vi "Toggle Debugging_Item_OnCommand.vi"(10 "Command ID":string, 11 "Object":T1) -> ()   [LabVIEW 2019]
uses:
  <resource>/Framework/Providers/API/ItemRef.ctl
panel:
  out "error out":errorcluster
  in  "error in":errorcluster
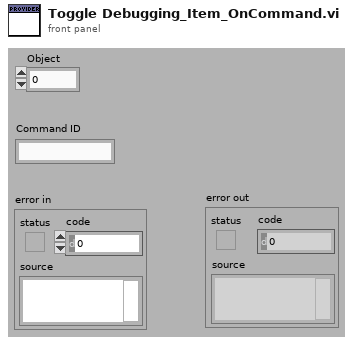
[diagram p1: front panel]
types:
  T1 = typedef "ItemRef.ctl" = u64
  T2 = enum32{"Invalid", "Standard", "Closed", "Hidden", "Minimized", "Maximized"}
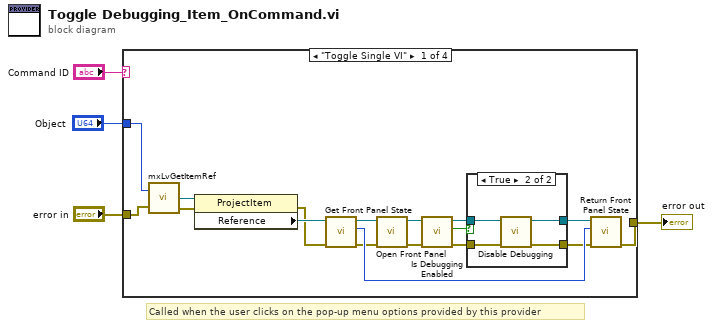
[diagram p0: block diagram]
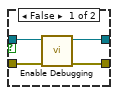
[diagram p2: hidden frame]
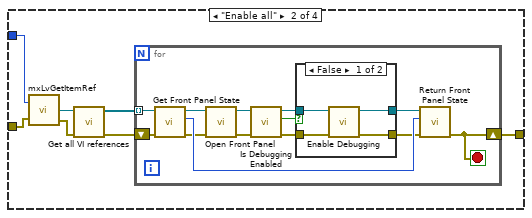
[diagram p3: hidden frame]
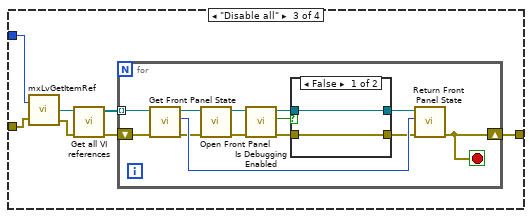
[diagram p5: hidden frame]
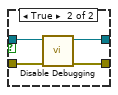
[diagram p6: hidden frame]
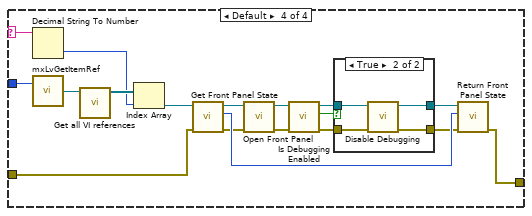
[diagram p7: hidden frame]
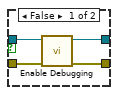
[diagram p8: hidden frame]
diagram:
  # "Called when the user clicks on the pop-up menu options provided by this provider"
  n1 = case shown="\"Toggle Single VI\"" "Command ID" {
    selector: "Command ID" -> [_ _ _ w99]
    tunnel: "error in" -> [w17 w32 w58 w83]
    tunnel: [w5 w30 w56 w82] -> w3
    tunnel: "Object" -> [w21 w35 w61 w98]
    frame "Toggle Single VI" {
      n2 = call <resource>:"mxLvGetItemRef.vi"("Item"=w21, "error in"=w17) -> ("Item Refnum"=w20:refnum<vi>, "error out"=w16:errorcluster)  [unwired: 1 out]
      n3 = property class="ProjectItem"(reference=w20, error in=w16) -> (error out=w8:errorcluster, "Reference"=w13:refnum<vi>)  [unwired: 1 out]
      n4 = call "Get Front Panel State.vi"("error in (no error)"=w8, "reference"=w13) -> ("error out"=w7:errorcluster, "Front Panel Window State"=w10:T2, "reference out"=w12:refnum<vi>)  [unwired: 7 in]
      n5 = call "Open Front Panel.vi"("error in (no error)"=w7, "reference"=w12) -> ("error out"=w6:errorcluster, "reference out"=w14:refnum<vi>)  [unwired: 8 in]
      n6 = call "Is Debugging Enabled.vi"("error in (no error)"=w6, "VI Reference In"=w14) -> ("error out"=w15:errorcluster, "Debugging Enabled?"=w19:bool, "VI Reference Out"=w18:refnum<vi>)  [unwired: 7 in]
      n7 = case shown="True" w19 {
        tunnel: w18 -> [w25 w29]
        tunnel: w15 -> [w24 w28]
        tunnel: [w23 w27] -> w9
        tunnel: [w22 w26] -> w11
        frame False {
          n8 = call "Enable Debugging.vi"("error in (no error)"=w24, "VI Reference In"=w25) -> ("error out"=w23:errorcluster, "VI Reference Out"=w22:refnum<vi>)  [unwired: 8 in]
        }
        frame True {
          n9 = call "Disable Debugging.vi"("error in (no error)"=w28, "VI Reference In"=w29) -> ("error out"=w27:errorcluster, "VI Reference Out"=w26:refnum<vi>)  [unwired: 8 in]
        }
      }
      n10 = call "Return Front Panel State.vi"("error in (no error)"=w9, "State"=w10, "reference"=w11) -> ("error out"=w5:errorcluster)  [unwired: 7 in, 1 out]
    }
    frame "Enable all" {
      n11 = call <resource>:"mxLvGetItemRef.vi"("Item"=w35, "error in"=w32) -> ("Item Refnum"=w36:refnum<vi>, "error out"=w33:errorcluster)  [unwired: 1 out]
      n12 = call "Get all VI references.vi"("error in (no error)"=w33, "Project Item"=w36) -> ("error out"=w31:errorcluster, "VI Refs"=w34:refnum<vi>[])  [unwired: 8 in]
      n13 = for {
        tunnel: w34 -> [w39] mode=indexing
        shift-right: [w37] -> w30
        shift-left: w31 -> [w38]
        stop <- w37 stop-if-true
        n14 = call "Get Front Panel State.vi"("error in (no error)"=w38, "reference"=w39) -> ("error out"=w41:errorcluster, "Front Panel Window State"=w43:T2, "reference out"=w45:refnum<vi>)  [unwired: 7 in]
        n15 = call "Open Front Panel.vi"("error in (no error)"=w41, "reference"=w45) -> ("error out"=w40:errorcluster, "reference out"=w46:refnum<vi>)  [unwired: 8 in]
        n16 = call "Is Debugging Enabled.vi"("error in (no error)"=w40, "VI Reference In"=w46) -> ("error out"=w47:errorcluster, "Debugging Enabled?"=w49:bool, "VI Reference Out"=w48:refnum<vi>)  [unwired: 7 in]
        n17 = case shown="False" w49 {
          tunnel: w48 -> [w53 w55]
          tunnel: w47 -> [w52 w54]
          tunnel: [w51 w54] -> w42
          tunnel: [w50 w55] -> w44
          frame False {
            n18 = call "Enable Debugging.vi"("error in (no error)"=w52, "VI Reference In"=w53) -> ("error out"=w51:errorcluster, "VI Reference Out"=w50:refnum<vi>)  [unwired: 8 in]
          }
          frame True {
          }
        }
        n19 = call "Return Front Panel State.vi"("error in (no error)"=w42, "State"=w43, "reference"=w44) -> ("error out"=w37:errorcluster)  [unwired: 7 in, 1 out]
      }
    }
    frame "Disable all" {
      n20 = call <resource>:"mxLvGetItemRef.vi"("Item"=w61, "error in"=w58) -> ("Item Refnum"=w62:refnum<vi>, "error out"=w59:errorcluster)  [unwired: 1 out]
      n21 = call "Get all VI references.vi"("error in (no error)"=w59, "Project Item"=w62) -> ("error out"=w57:errorcluster, "VI Refs"=w60:refnum<vi>[])  [unwired: 8 in]
      n22 = for {
        tunnel: w60 -> [w65] mode=indexing
        shift-right: [w63] -> w56
        shift-left: w57 -> [w64]
        stop <- w63 stop-if-true
        n23 = call "Get Front Panel State.vi"("error in (no error)"=w64, "reference"=w65) -> ("error out"=w67:errorcluster, "Front Panel Window State"=w69:T2, "reference out"=w71:refnum<vi>)  [unwired: 7 in]
        n24 = call "Open Front Panel.vi"("error in (no error)"=w67, "reference"=w71) -> ("error out"=w66:errorcluster, "reference out"=w72:refnum<vi>)  [unwired: 8 in]
        n25 = call "Is Debugging Enabled.vi"("error in (no error)"=w66, "VI Reference In"=w72) -> ("error out"=w73:errorcluster, "Debugging Enabled?"=w75:bool, "VI Reference Out"=w74:refnum<vi>)  [unwired: 7 in]
        n26 = case shown="False" w75 {
          tunnel: w74 -> [w77 w81]
          tunnel: w73 -> [w76 w80]
          tunnel: [w76 w79] -> w68
          tunnel: [w77 w78] -> w70
          frame False {
          }
          frame True {
            n27 = call "Disable Debugging.vi"("error in (no error)"=w80, "VI Reference In"=w81) -> ("error out"=w79:errorcluster, "VI Reference Out"=w78:refnum<vi>)  [unwired: 8 in]
          }
        }
        n28 = call "Return Front Panel State.vi"("error in (no error)"=w68, "State"=w69, "reference"=w70) -> ("error out"=w63:errorcluster)  [unwired: 7 in, 1 out]
      }
    }
    frame Default {
      n29 = Decimal String To Number(string=w99) -> (number=w95:i32)  [unwired: 2 in, 1 out]
      n30 = call <resource>:"mxLvGetItemRef.vi"("Item"=w98) -> ("Item Refnum"=w97:refnum<vi>)  [unwired: 1 in, 2 out]
      n31 = call "Get all VI references.vi"("Project Item"=w97) -> ("VI Refs"=w96:refnum<vi>[])  [unwired: 9 in, 1 out]
      n32 = Index Array(array=w96, index=w95) -> (element=w84:refnum<vi>)
      n33 = call "Get Front Panel State.vi"("error in (no error)"=w83, "reference"=w84) -> ("error out"=w86:errorcluster, "Front Panel Window State"=w88:T2, "reference out"=w90:refnum<vi>)  [unwired: 7 in]
      n34 = call "Open Front Panel.vi"("error in (no error)"=w86, "reference"=w90) -> ("error out"=w85:errorcluster, "reference out"=w91:refnum<vi>)  [unwired: 8 in]
      n35 = call "Is Debugging Enabled.vi"("error in (no error)"=w85, "VI Reference In"=w91) -> ("error out"=w92:errorcluster, "Debugging Enabled?"=w94:bool, "VI Reference Out"=w93:refnum<vi>)  [unwired: 7 in]
      n36 = case shown="True" w94 {
        tunnel: w93 -> [w103 w107]
        tunnel: w92 -> [w102 w106]
        tunnel: [w101 w105] -> w87
        tunnel: [w100 w104] -> w89
        frame False {
          n37 = call "Enable Debugging.vi"("error in (no error)"=w102, "VI Reference In"=w103) -> ("error out"=w101:errorcluster, "VI Reference Out"=w100:refnum<vi>)  [unwired: 8 in]
        }
        frame True {
          n38 = call "Disable Debugging.vi"("error in (no error)"=w106, "VI Reference In"=w107) -> ("error out"=w105:errorcluster, "VI Reference Out"=w104:refnum<vi>)  [unwired: 8 in]
        }
      }
      n39 = call "Return Front Panel State.vi"("error in (no error)"=w87, "State"=w88, "reference"=w89) -> ("error out"=w82:errorcluster)  [unwired: 7 in, 1 out]
    }
  }
  "error out" <- w3
